vi "产生序列.vi"(1 "码速率RB":dbl, 2 "采样率":dbl, 3 "输入序列":u32[](array[numeric]) format="%b") -> (0 "输入序列波形":dbl[](array[numeric]))   [LabVIEW 2011]
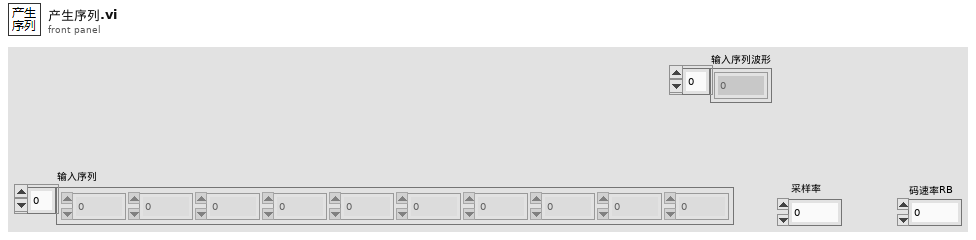
[diagram p1: front panel]
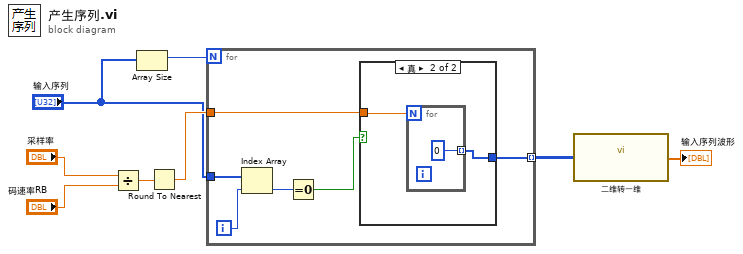
[diagram p0: block diagram]
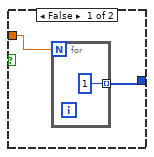
[diagram p2: hidden frame]
diagram:
  n1 = Divide(x="采样率", y="码速率RB") -> (x/y=w6:dbl)
  n2 = Array Size(array="输入序列") -> (size(s)=w5:i32)
  n3 = Round To Nearest(number=w6) -> (nearest integer value=w4:dbl)
  n4 = for {
    N: w5 -> [_]
    tunnel: w4 -> [w10]
    tunnel: "输入序列" -> [w13]
    tunnel: [w9] -> w2 mode=indexing
    i -> [w14]
    n5 = Index Array(array=w13, index=w14) -> (element=w12:u32)
    n6 = Equal To 0?(x=w12) -> (x = 0?=w11:bool)
    n7 = case shown="真" w11 {
      tunnel: w10 -> [w16 w19]
      tunnel: [w15 w18] -> w9
      frame False {
        n8 = for {
          N: w16 -> [_]
          tunnel: [1] -> w15 mode=indexing
        }
      }
      frame True {
        n9 = for {
          N: w19 -> [_]
          tunnel: [0] -> w18 mode=indexing
        }
      }
    }
  }
  n10 = call "二维转一维.vi"("输入2维"=w2) -> ("输出一维"=→"输入序列波形":dbl[])
